vi "FMSweep-Compute Max Level.vi"(0 "FMSweep":T3, 9 "Level":T1, 11 "error in (no error)":errorcluster, 12 "Fs (Hz)":dbl) -> (6 "Max Level":dbl, 10 "Level out":T1, 15 "error out":errorcluster)   [LabVIEW 2020]
uses:
  FM Sweep Params.ctl
  Controls/Level XCtl/Level Data.ctl
  Controls/Level XCtl/Level Units.ctl
  <vilib>/Analysis/baseanly.llb/Mean (DBL).vi
  Utility VIs/Math VIs/Linear to dB (scalar).vi
  PXI DAQ VIs/DAQ Engine VIs/PXI Globals.vi
  <vilib>/Analysis/NI_AALBase.lvlib
  Controls/Level XCtl/Level XCtl.xctl
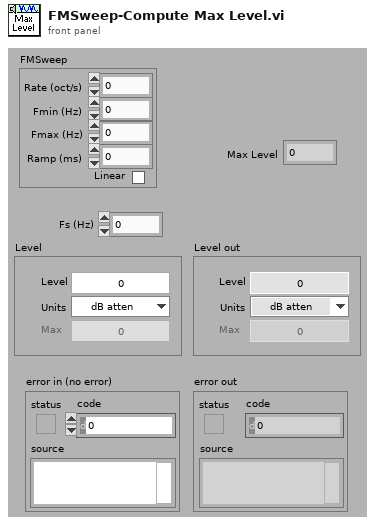
[diagram p1: front panel]
types:
  T1 = typedef "Level XCtl.xctl/Level Data.ctl" = cluster{"Level":dbl, "Units":T2, "Max":dbl, "Multiplier":dbl, "Cal File":path, "Cal":cluster{"Freq (Hz)":dbl[], "Mag (dB SPL)":dbl[], "Phase (deg)":dbl[]}}
  T2 = typedef "Level Units.ctl" = enum16{"dB atten", "dB SPL", "dB re 1 Vrms", "dB V/Hz½", "mW", "dB HL", "Volts", "dB mW"}
  T3 = typedef "FM Sweep Params.ctl" = cluster{"Rate (oct/s)":dbl, "Fmin (Hz)":dbl, "Fmax (Hz)":dbl, "Ramp (ms)":dbl, "Linear":bool}
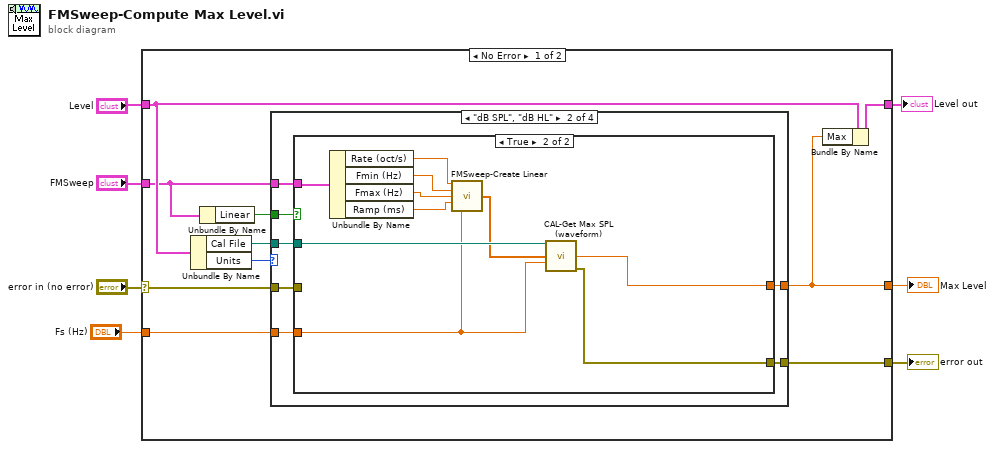
[diagram p0: block diagram]
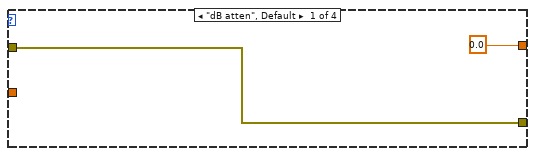
[diagram p2: hidden frame]
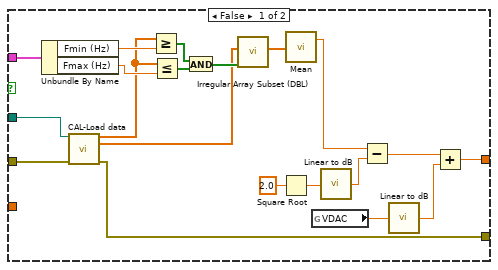
[diagram p3: hidden frame]
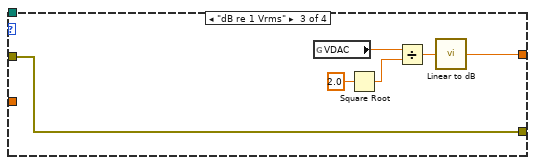
[diagram p4: hidden frame]
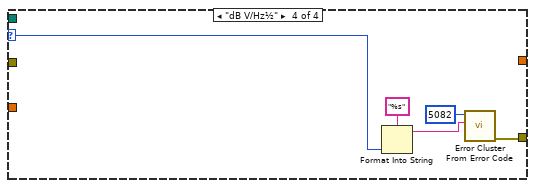
[diagram p5: hidden frame]
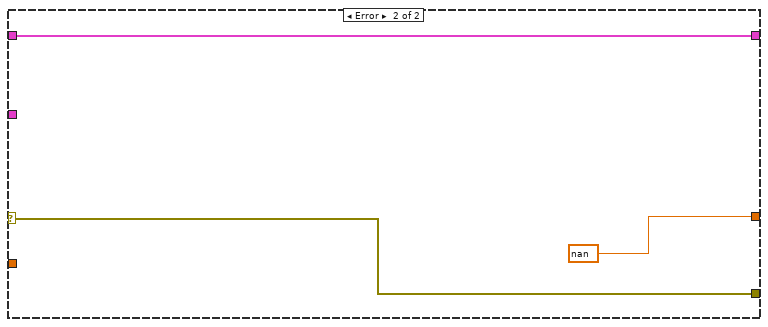
[diagram p6: hidden frame]
diagram:
  n1 = case shown="No Error" "error in (no error)" {
    selector: "error in (no error)" -> [w17 w70]
    tunnel: "Level" -> [w15 w68]
    tunnel: "FMSweep" -> [w10 _]
    tunnel: [w16 w70] -> w6
    tunnel: [w14 nan ("Reference Level")] -> w3
    tunnel: [w13 w68] -> w2
    tunnel: "Fs (Hz)" -> [w8 _]
    frame No Error {
      n2 = Unbundle By Name(w15) -> ("Cal File"=w12:path, "Units"=w11:T2)
      n3 = Unbundle By Name(w10) -> ("Linear"=w9:bool)
      n4 = case shown="\"dB SPL\", \"dB HL\"" w11 {
        selector: w11 -> [_ _ _ w63]
        tunnel: w17 -> [w18 w26 w62 _]
        tunnel: w10 -> [_ w24 _ _]
        tunnel: [0.0 ("Reference Level") w25 w57 _] -> w14
        tunnel: [w18 w23 w62 w64] -> w16
        tunnel: w12 -> [_ w22 _ _]
        tunnel: w9 -> [_ w21 _ _]
        tunnel: w8 -> [_ w20 _ _]
        frame "dB atten", Default {
        }
        frame "dB SPL", "dB HL" {
          n5 = case shown="True" w21 {
            tunnel: w26 -> [w46 _]
            tunnel: [w44 w48] -> w25
            tunnel: w24 -> [w41 w55]
            tunnel: [w37 w47] -> w23
            tunnel: w22 -> [w36 w56]
            tunnel: w20 -> [_ w50]
            frame False {
              n6 = Unbundle By Name(w41) -> ("Fmin (Hz)"=w35:dbl, "Fmax (Hz)"=w34:dbl)
              n7 = call "CAL-Load data.vi"("user path"=w36, "error in (no error)"=w46) -> ("Frequency (Hz)"=w33:dbl[], "Mag"=w29:dbl[], "error out"=w37:errorcluster)  [unwired: 6 in, 5 out]
              n8 = Greater Or Equal?(x=w33, y=w35) -> (x >= y?=w32:bool[])
              n9 = Less Or Equal?(x=w33, y=w34) -> (x <= y?=w31:bool[])
              n10 = And(x=w32, y=w31) -> (x .and. y?=w30:bool[])
              n11 = call "Irregular Array Subset (DBL).vi"("Mask"=w30, "Array"=w29) -> ("Array Subset"=w28:dbl[])  [unwired: 8 in, 1 out]
              n12 = Square Root(x=2.0 ("y")) -> (sqrt(x)=w40:dbl)
              n13 = call-poly <vilib>:"Mean.vi"("X"=w28) -> ("mean"=w27:dbl)  [unwired: 1 out]
              n14 = global read "PXI Globals.vi" "VDAC"() -> (w45:dbl)
              n15 = call-poly "Linear to dB.vi"("Linear"=w40) -> ("dB"=w39:dbl)
              n16 = Subtract(x=w27, y=w39) -> (x-y=w38:dbl)
              n17 = call-poly "Linear to dB.vi"("Linear"=w45) -> ("dB"=w43:dbl)
              n18 = Add(x=w38, y=w43) -> (x+y=w44:dbl)
            }
            frame True {
              n19 = Unbundle By Name(w55) -> ("Rate (oct/s)"=w54:dbl, "Fmin (Hz)"=w53:dbl, "Fmax (Hz)"=w52:dbl, "Ramp (ms)"=w51:dbl)
              n20 = call "FMSweep-Create Linear.vi"("Sweep Rate (Hz/s)"=w54, "Fmin (Hz)"=w53, "Fmax (Hz)"=w52, "Ramp (ms)"=w51, "Fs (Hz)"=w50) -> ("Array"=w49:dbl[])  [unwired: 8 in, 2 out]
              n21 = call "CAL-Get Max SPL (waveform).vi"("Cal File"=w56, "Y"=w49, "Sampling Rate (Hz)"=w50) -> ("Max SPL"=w48:dbl, "error out"=w47:errorcluster)  [unwired: 11 in]
            }
          }
        }
        frame "dB re 1 Vrms" {
          n22 = global read "PXI Globals.vi" "VDAC"() -> (w59:dbl)
          n23 = Square Root(x=2.0 ("y")) -> (sqrt(x)=w60:dbl)
          n24 = Divide(x=w59, y=w60) -> (x/y=w58:dbl)
          n25 = call-poly "Linear to dB.vi"("Linear"=w58) -> ("dB"=w57:dbl)
        }
        frame "dB V/Hz½" {
          n26 = Format Into String(format string="%s", w63) -> (resulting string=w66:string)  [unwired: 2 in, 1 out]
          n27 = call <vilib>:"Error Cluster From Error Code.vi"("error message (\"\")"=w66, "error code (0)"=5082) -> ("error out"=w64:errorcluster)  [unwired: 7 in]
        }
      }
      n28 = Bundle By Name(cluster=w15, "Max"=w14) -> (w13:T1)
    }
    frame Error {
    }
  }
  "error out" <- w6
  "Max Level" <- w3
  "Level out" <- w2
